vi "Label Caption Visible write.vi"(7 "Caption.Visible":bool, 8 "Label.Visible":bool, 9 "Ctl Refnum in":refnum<vi>) -> (3 "Ctl Refnum out":refnum<vi>)   [LabVIEW 2010, in "Control.lvclass"]
uses:
  Control.lvclass
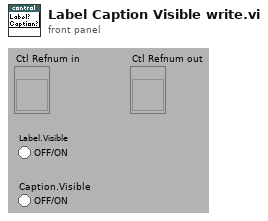
[diagram p1: front panel]
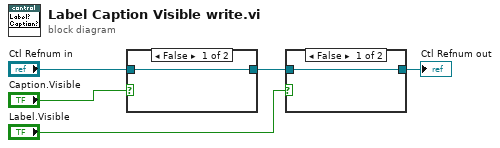
[diagram p0: block diagram]
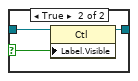
[diagram p2: hidden frame]
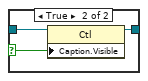
[diagram p3: hidden frame]
diagram:
  n1 = case shown="False" "Caption.Visible" {
    selector: "Caption.Visible" -> [_ w7]
    tunnel: "Ctl Refnum in" -> [w6 w9]
    tunnel: [w6 w8] -> w2
    frame False {
    }
    frame True {
      n2 = property class="Ctl"(reference=w9, "Caption.Visible"=w7) -> (reference out=w8:refnum<vi>)  [unwired: 1 in, 1 out]
    }
  }
  n3 = case shown="False" "Label.Visible" {
    selector: "Label.Visible" -> [_ w11]
    tunnel: w2 -> [w10 w13]
    tunnel: [w10 w12] -> w4
    frame False {
    }
    frame True {
      n4 = property class="Ctl"(reference=w13, "Label.Visible"=w11) -> (reference out=w12:refnum<vi>)  [unwired: 1 in, 1 out]
    }
  }
  "Ctl Refnum out" <- w4
